vi "SetQbusRef_FGV.vi"(8 "error in (no error)":errorcluster, 11 "Qbus in":refnum<class "Qbus.lvclass">) -> (0 "error out":errorcluster, 3 "Qbus out":refnum<class "Qbus.lvclass">)   [LabVIEW 2017, in "Qbus.lvclass"]
uses:
  <vilib>/addons/Qbus/Qbus.lvclass
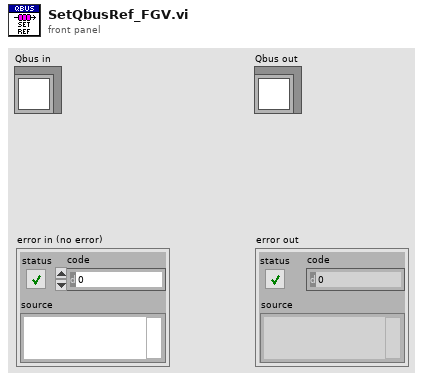
[diagram p1: front panel]
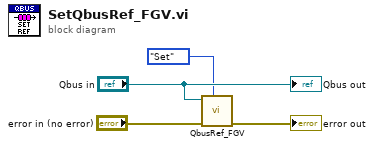
[diagram p0: block diagram]
diagram:
  n1 = call <vilib>:"QbusRef_FGV.vi"("action"=enum16{"Set", "Get"}."Set" ("Action"), "error in (no error)"="error in (no error)", "Qbus in"="Qbus in") -> ("error out"=→"error out":errorcluster)  [unwired: 7 in, 1 out]
  "Qbus out" <- "Qbus in"
